vi "Update PGconn and PGResults type.vi"(10 "Numeric Type":T2(ring), 11 "ParamInfo":T1(array[cluster])) -> (2 "Change":bool, 3 "ParamInfo":T1(array[cluster]))   [LabVIEW 2017]
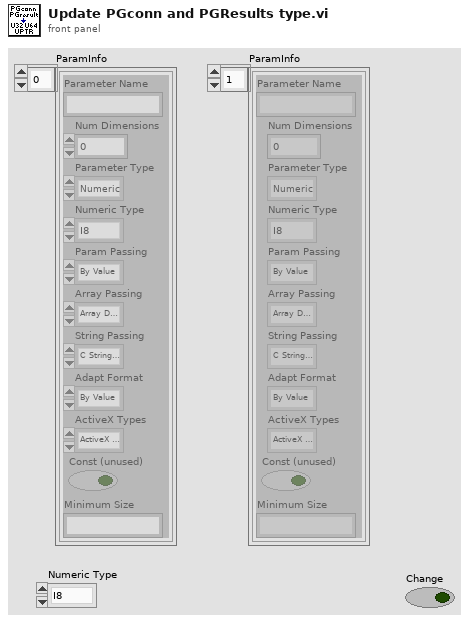
[diagram p1: front panel]
types:
  T1 = cluster{"Parameter Name":string, "Num Dimensions":i32, "Parameter Type":enum16{"Numeric", "Array", "String", "Waveform", "Digital Waveform", "Digital Table", "ActiveX", "Any", "Instance Data Pointer", "Void"}, "Numeric Type":enum16{"I8", "I16", "I32", "I64", "U8", "U16", "U32", "U64", "SGL", "DBL", "PTR INT", "PTR UINT"}, "Param Passing":enum16{"By Value", "Pointer To Value"}, "Array Passing":enum16{"Array Data Pointer", "Array Handle", "Array Handle Pointer"}, "String Passing":enum16{"C String Pointer", "Pascal String Pointer", "String Handle", "String Handle Pointer"}, "Adapt Format":enum16{"By Value", "Pointer To Value"}, "ActiveX Types":enum16{"ActiveX Variant Pointer", "IDispatch* Pointer", "IUnknown* Pointer"}, "Const (unused)":bool, "Minimum Size":string}[]
  T2 = enum16{"I8", "I16", "I32", "I64", "U8", "U16", "U32", "U64", "SGL", "DBL", "PTR INT", "PTR UINT"}
  T3 = cluster{"Parameter Name":string, "Num Dimensions":i32, "Parameter Type":enum16{"Numeric", "Array", "String", "Waveform", "Digital Waveform", "Digital Table", "ActiveX", "Any", "Instance Data Pointer", "Void"}, "Numeric Type":enum16{"I8", "I16", "I32", "I64", "U8", "U16", "U32", "U64", "SGL", "DBL", "PTR INT", "PTR UINT"}, "Param Passing":enum16{"By Value", "Pointer To Value"}, "Array Passing":enum16{"Array Data Pointer", "Array Handle", "Array Handle Pointer"}, "String Passing":enum16{"C String Pointer", "Pascal String Pointer", "String Handle", "String Handle Pointer"}, "Adapt Format":enum16{"By Value", "Pointer To Value"}, "ActiveX Types":enum16{"ActiveX Variant Pointer", "IDispatch* Pointer", "IUnknown* Pointer"}, "Const (unused)":bool, "Minimum Size":string}
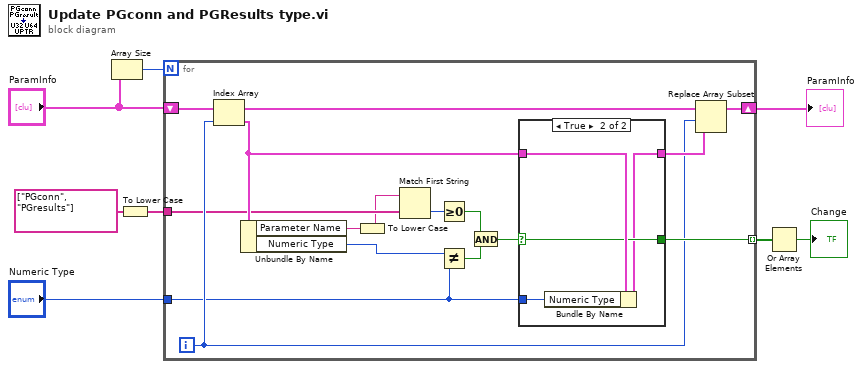
[diagram p0: block diagram]
diagram:
  n1 = Array Size(array="ParamInfo") -> (size(s)=w4:i32)
  n2 = To Lower Case(string=string[] ["PGconn", "PGresults"] ("x")) -> (all lower case string=w1:string[])
  n3 = for {
    N: w4 -> [_]
    tunnel: [w23] -> w7 mode=indexing
    shift-right: [w20] -> w6
    shift-left: "ParamInfo" -> [w21]
    tunnel: w1 -> [w14]
    tunnel: "Numeric Type" -> [w15]
    i -> [w18]
    n4 = Index Array(array=w21, index=w18) -> (element=w22:T3)
    n5 = Unbundle By Name(w22) -> ("Parameter Name"=w13:string, "Numeric Type"=w10:T2)
    n6 = To Lower Case(string=w13) -> (all lower case string=w9:string)
    n7 = Match First String(2:w14, 3:w9) -> (0:w12:i32)  [unwired: 1 out]
    n8 = Greater Or Equal To 0?(x=w12) -> (x >= 0?=w11:bool)
    n9 = Not Equal?(x=w10, y=w15) -> (x != y?=w17:bool)
    n10 = And(x=w11, y=w17) -> (x .and. y?=w16:bool)
    n11 = case shown="True" w16 {
      selector: w16 -> [w25 w28]
      tunnel: w22 -> [w24 w29]
      tunnel: [w25 w28] -> w23
      tunnel: [w24 w27] -> w19
      tunnel: w15 -> [_ w26]
      frame False {
      }
      frame True {
        n12 = Bundle By Name(cluster=w29, "Numeric Type"=w26) -> (w27:T3)
      }
    }
    n13 = Replace Array Subset(array=w21, new element=w19, index=w18) -> (w20:T1)
  }
  "ParamInfo" <- w6
  n14 = Or Array Elements(Boolean array=w7) -> (logical OR=→"Change":bool)
